vi "saving images.vi"() -> ()   [LabVIEW 2018]
uses:
  <vilib>/picture/picture.llb/imagedata.ctl
panel:
  in  "new picture":picture
  in  "path to JPEG file 2":path
  in  "image data 2":T1
  in  "path to JPEG file":path
  out "image data":T1
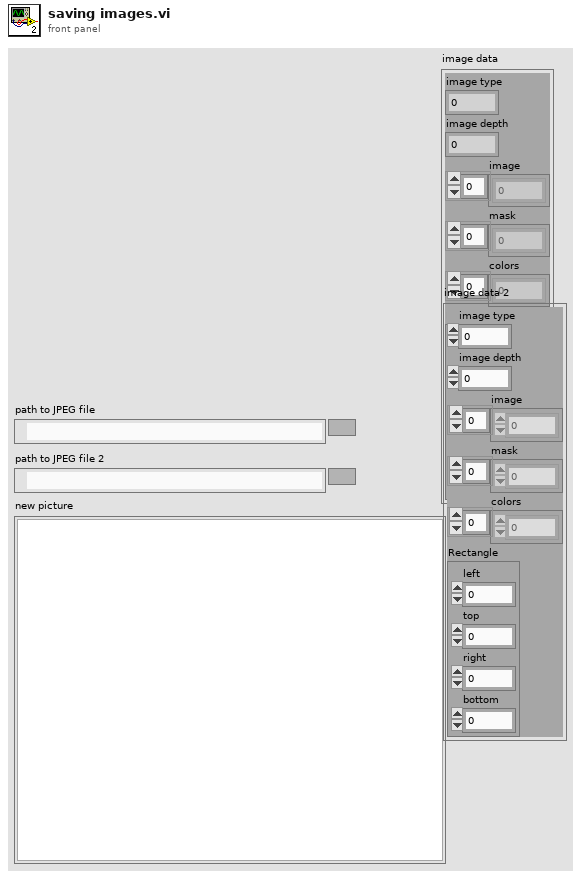
[diagram p1: front panel]
types:
  T1 = typedef "imagedata.ctl" = cluster{"image type":i32, "image depth":i32, "image":u8[], "mask":u8[], "colors":u32[], "Rectangle":cluster{"left":i16, "top":i16, "right":i16, "bottom":i16}}
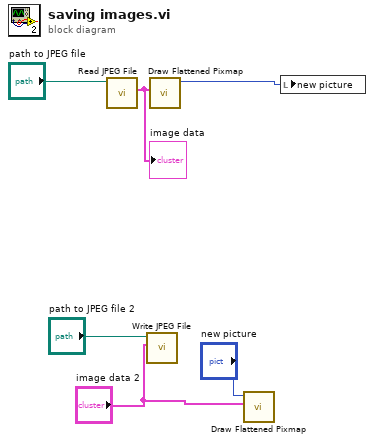
[diagram p0: block diagram]
diagram:
  n1 = call <vilib>:"Read JPEG File.vi"("path to JPEG file"="path to JPEG file") -> ("image data"=w6:T1)  [unwired: 8 in, 2 out]
  "image data" <- w6
  n2 = call <vilib>:"Write JPEG File.vi"("image data"="image data 2", "path to JPEG file"="path to JPEG file 2") -> ()  [unwired: 8 in, 2 out]
  n3 = call <vilib>:"Draw Flattened Pixmap.vi"("image data"=w6) -> ("new picture"=w1:picture)  [unwired: 8 in]
  n4 = call <vilib>:"Draw Flattened Pixmap.vi"("image data"="image data 2", "picture"="new picture") -> ()  [unwired: 7 in, 1 out]
  n5 = local write "new picture"(w1) -> ()
